vi "Validate Transmit SubAddress.vi"(4 "RT Address (0-30)":u8, 6 "RT 1?":bool, 8 "error in (no error)":errorcluster, 11 "1553 Unit Test in":refnum<class "Remote Terminal.lvclass">) -> (0 "error out":errorcluster, 3 "1553 Unit Test out":refnum<class "Remote Terminal.lvclass">)   [LabVIEW 2020, in "Unit Tests.lvlib" / "Remote Terminal.lvclass"]
uses:
  Remote Terminal.lvclass
  Remote Terminal.lvclass/Remote Terminal.ctl
  <vilib>/addons/_JKI Toolkits/Caraya/classes/Assert/Assert True.vi
  Dependencies/FPGA Interface/FPGA Interface.lvclass
  <vilib>/addons/_JKI Toolkits/Caraya/classes/Assert/Assert.lvclass
  <vilib>/addons/_JKI Toolkits/Caraya/classes/Test/Test.lvclass
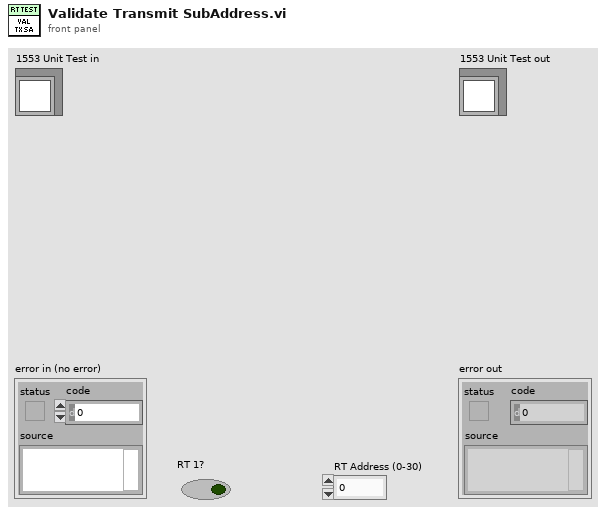
[diagram p1: front panel]
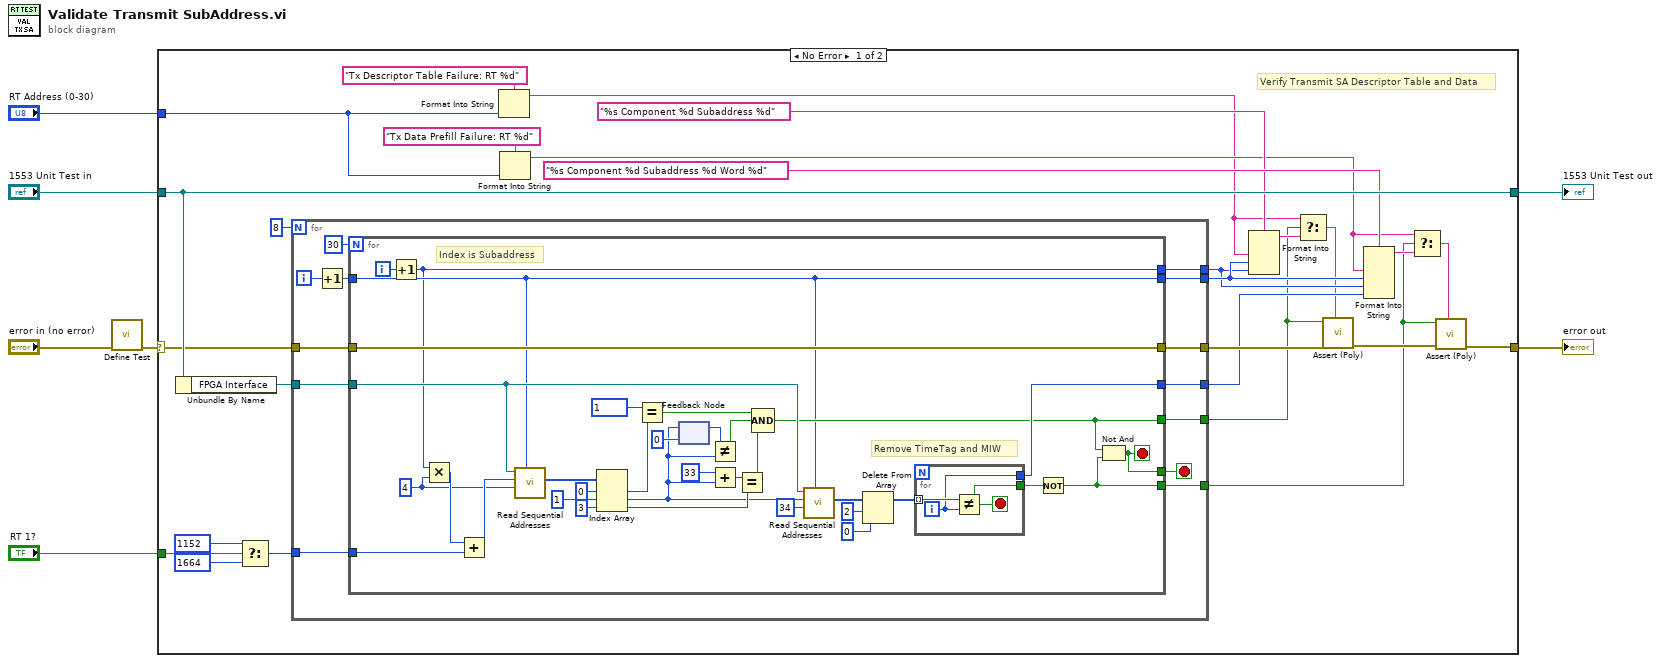
[diagram p0: block diagram]
diagram:
  n1 = call <vilib>:"Define Test.vi"("error in (no error)"="error in (no error)") -> ("error out"=w3:errorcluster)  [unwired: 9 in, 1 out]
  n2 = case shown="No Error" w3 {
    selector: w3 -> [w27 w86]
    tunnel: [w24 w86] -> w7
    tunnel: [w29 w85] -> w5
    tunnel: "1553 Unit Test in" -> [w29 w85]
    tunnel: "RT 1?" -> [w32 _]
    tunnel: "RT Address (0-30)" -> [w9 _]
    frame No Error {
      # "Verify Transmit SA Descriptor Table and Data"
      n3 = Unbundle By Name(w29) -> ("FPGA Interface"=w28:refnum<class "FPGA Interface.lvclass">)
      n4 = Select(t=u16 1152, s=w32, f=u16 1664) -> (s? t:f=w30:u16)
      n5 = for {
        N: 8 -> [_]
        tunnel: w30 -> [w35]
        tunnel: w28 -> [w44]
        tunnel: [w43] -> w26
        tunnel: w27 -> [w42]
        tunnel: [w37] -> w11
        tunnel: [w38] -> w15
        tunnel: [w41] -> w19
        tunnel: [w40] -> w20
        tunnel: [w39] -> w18
        i -> [w47]
        stop <- w36 stop-if-true
        n6 = Increment(x=w47) -> (x+1=w45:i32)
        n7 = for {
          N: 30 -> [_]
          tunnel: w45 -> [w53]
          tunnel: w44 -> [w81]
          tunnel: [w80] -> w43
          tunnel: w42 -> [w80]
          tunnel: [w77] -> w37
          tunnel: [w78] -> w38
          tunnel: [w52] -> w41
          tunnel: [w53] -> w40
          tunnel: [w79] -> w39
          tunnel: [w76] -> w36
          tunnel: w35 -> [w50]
          i -> [w54]
          stop <- w76 stop-if-true
          w48 = u16 4 ("x")
          # "Index is Subaddress"
          # "Remove TimeTag and MIW"
          n8 = Increment(x=w54) -> (x+1=w52:i32)
          n9 = Multiply(x=w52, y=w48) -> (x*y=w51:i32)
          n10 = Add(x=w51, y=w50) -> (x+y=w49:i32)
          n11 = call-dynamic "Read Sequential Addresses.vi"("Target IC (1-8)"=w53, "Addresses to Read"=w48, "Starting Address"=w49, "FPGA Interface in"=w81) -> ("Data"=w62:u16[])  [unwired: 6 in, 1 out]
          n12 = Index Array(array=w62, index #1=0 ("index"), index #2=1 ("index"), index #3=3 ("index")) -> (element #1=w68:u16, element #2=w61:u16, element #3=w64:u16)
          n13 = Equal?(x=u16 1, y=w68) -> (x = y?=w71:bool)
          n14 = feedback #1(u16 0 ("Data")) -> (w70:u16)
          n15 = feedback-in #1(w61) -> ()
          n16 = Not Equal?(x=w70, y=w61) -> (x != y?=w69:bool)
          n17 = Add(x=u16 33, y=w61) -> (x+y=w66:u16)
          n18 = Equal?(x=w66, y=w64) -> (x = y?=w65:bool)
          n19 = Compound Arithmetic op=AND(w71, w69, w65) -> (w78:bool)
          n20 = call-dynamic "Read Sequential Addresses.vi"("Target IC (1-8)"=w53, "Addresses to Read"=u16 34, "Starting Address"=w61, "FPGA Interface in"=w81) -> ("Data"=w56:u16[])  [unwired: 6 in, 1 out]
          n21 = Delete From Array(array=w56, length=2, index=0) -> (array with subset deleted=w59:u16[])  [unwired: 1 out]
          n22 = for {
            tunnel: w59 -> [w84] mode=indexing
            tunnel: [w83] -> w55
            tunnel: [w82] -> w79
            i -> [w82]
            stop <- w83 stop-if-true
            n23 = Not Equal?(x=w84, y=w82) -> (x != y?=w83:bool)
          }
          n24 = Not(x=w55) -> (.not. x?=w77:bool)
          n25 = Not And(1:w77, 2:w78) -> (0:w76:bool)
        }
      }
      n26 = Format Into String(format string="Tx Descriptor Table Failure: RT %d" ("message (\"\")"), w9) -> (resulting string=w8:string)  [unwired: 2 in, 1 out]
      n27 = Format Into String(format string="Tx Data Prefill Failure: RT %d" ("message (\"\")"), w9) -> (resulting string=w12:string)  [unwired: 2 in, 1 out]
      n28 = Format Into String(format string="%s Component %d Subaddress %d" ("message (\"\")"), w8, w20, w19) -> (resulting string=w17:string)  [unwired: 2 in, 1 out]
      n29 = Select(t=w8, s=w15, f=w17) -> (s? t:f=w14:string)
      n30 = call-poly <vilib>:"Assert (Poly).vi"("Label"=w14, "error in (no error)"=w26, "True?"=w15) -> ("error out"=w25:errorcluster)  [unwired: 7 in, 1 out]
      n31 = Format Into String(format string="%s Component %d Subaddress %d Word %d" ("message (\"\")"), w12, w20, w19, w18) -> (resulting string=w13:string)  [unwired: 2 in, 1 out]
      n32 = Select(t=w12, s=w11, f=w13) -> (s? t:f=w10:string)
      n33 = call-poly <vilib>:"Assert (Poly).vi"("Label"=w10, "error in (no error)"=w25, "True?"=w11) -> ("error out"=w24:errorcluster)  [unwired: 7 in, 1 out]
    }
    frame Error {
    }
  }
  "error out" <- w7
  "1553 Unit Test out" <- w5
